vi "Sagar C V Comparator.vi"() -> ()   [LabVIEW 2018]
panel:
  in  "?":string
  in  "?":string
  out "A<B":bool
  out "A=B":bool
  out "A>B":bool
  in  "B0":bool
  in  "B1":bool
  in  "A0":bool
  in  "A1":bool
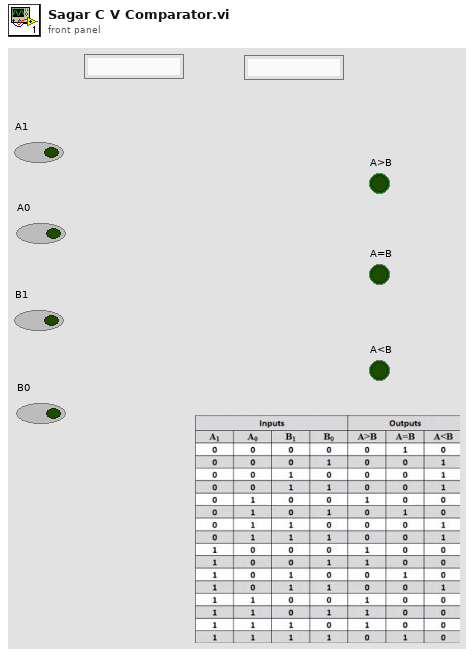
[diagram p1: front panel]
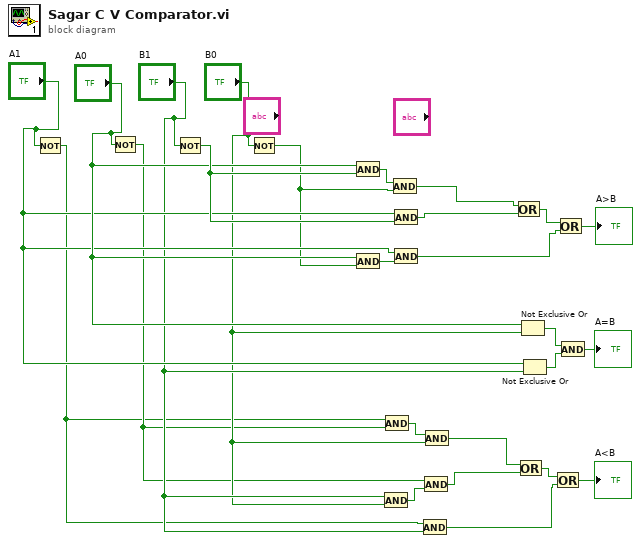
[diagram p0: block diagram]
diagram:
  n1 = Not(x="A1") -> (.not. x?=w1:bool)
  n2 = Not(x="A0") -> (.not. x?=w2:bool)
  n3 = Not(x="B1") -> (.not. x?=w15:bool)
  n4 = Not(x="B0") -> (.not. x?=w10:bool)
  n5 = And(x="A0", y=w15) -> (x .and. y?=w17:bool)
  n6 = And(x="A0", y=w10) -> (x .and. y?=w16:bool)
  n7 = And(x="B1", y="B0") -> (x .and. y?=w8:bool)
  n8 = And(x=w1, y=w2) -> (x .and. y?=w9:bool)
  n9 = And(x=w17, y=w10) -> (x .and. y?=w14:bool)
  n10 = And(x="A1", y=w15) -> (x .and. y?=w18:bool)
  n11 = And(x="A1", y=w16) -> (x .and. y?=w13:bool)
  n12 = And(x=w1, y="B1") -> (x .and. y?=w7:bool)
  n13 = And(x=w2, y=w8) -> (x .and. y?=w6:bool)
  n14 = And(x=w9, y="B0") -> (x .and. y?=w5:bool)
  n15 = Or(x=w14, y=w18) -> (x .or. y?=w24:bool)
  n16 = Or(x=w5, y=w6) -> (x .or. y?=w21:bool)
  n17 = Not Exclusive Or(1:"B0", 2:"A0") -> (0:w20:bool)
  n18 = Not Exclusive Or(1:"B1", 2:"A1") -> (0:w19:bool)
  n19 = Or(x=w21, y=w7) -> (x .or. y?=→"A<B":bool)
  n20 = Or(x=w24, y=w13) -> (x .or. y?=→"A>B":bool)
  n21 = And(x=w20, y=w19) -> (x .and. y?=→"A=B":bool)
